vi "(SubVI) Calculate all frame BM (mean10).vi"(10 "y position (pixel)":dbl[](array[numeric]), 11 "x position (pixel)":dbl[](array[numeric])) -> (0 "y standard deviation":dbl, 3 "x standard deviation":dbl, 4 "y position (delete y fit error)":dbl[](array[numeric]), 5 "x position (delete x fit error)":dbl[](array[numeric]))   [LabVIEW 2016]
uses:
  <vilib>/Analysis/NI_AALBase.lvlib
panel:
  out "y standard deviation 2":dbl
  out "x standard deviation 2":dbl
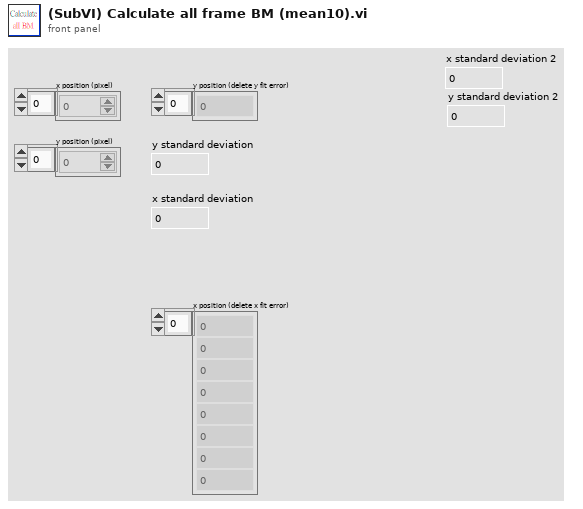
[diagram p1: front panel]
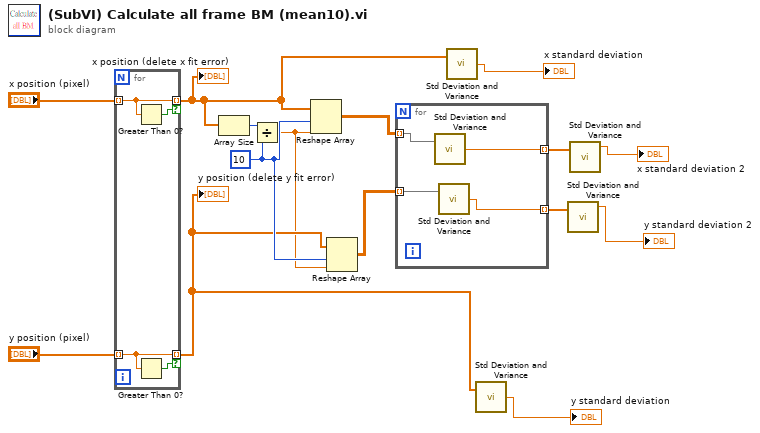
[diagram p0: block diagram]
diagram:
  w6 = 10 ("dimension size")
  n1 = for {
    tunnel: [w17] -> w5 mode=indexing if=w16
    tunnel: [w18] -> w11 mode=indexing if=w19
    tunnel: "x position (pixel)" -> [w18] mode=indexing
    tunnel: "y position (pixel)" -> [w17] mode=indexing
    n2 = Greater Than 0?(x=w18) -> (x > 0?=w19:bool)
    n3 = Greater Than 0?(x=w17) -> (x > 0?=w16:bool)
  }
  "y position (delete y fit error)" <- w5
  "x position (delete x fit error)" <- w11
  n4 = Array Size(array=w11) -> (size(s)=w10:i32)
  n5 = Divide(x=w10, y=w6) -> (x/y=w4:dbl)
  n6 = Reshape Array(w11, w6, w4) -> (w9:dbl[][])
  n7 = Reshape Array(w5, w6, w4) -> (w3:dbl[][])
  n8 = for {
    tunnel: w9 -> [w23] mode=indexing
    tunnel: [w22] -> w8 mode=indexing
    tunnel: w3 -> [w21] mode=indexing
    tunnel: [w20] -> w2 mode=indexing
    n9 = call <vilib>:"Std Deviation and Variance.vi"("X"=w23) -> ("standard deviation"=w22:dbl)  [unwired: 1 in, 2 out]
    n10 = call <vilib>:"Std Deviation and Variance.vi"("X"=w21) -> ("standard deviation"=w20:dbl)  [unwired: 1 in, 2 out]
  }
  n11 = call <vilib>:"Std Deviation and Variance.vi"("X"=w11) -> ("standard deviation"=→"x standard deviation":dbl)  [unwired: 1 in, 2 out]
  n12 = call <vilib>:"Std Deviation and Variance.vi"("X"=w5) -> ("standard deviation"=→"y standard deviation":dbl)  [unwired: 1 in, 2 out]
  n13 = call <vilib>:"Std Deviation and Variance.vi"("X"=w2) -> ("mean"=→"y standard deviation 2":dbl)  [unwired: 1 in, 2 out]
  n14 = call <vilib>:"Std Deviation and Variance.vi"("X"=w8) -> ("mean"=→"x standard deviation 2":dbl)  [unwired: 1 in, 2 out]
